vi "Rotation Matrix to Transform.vi"(1 "translation vector":dbl[](array[numeric]), 2 "rotation matrix":T1=[[1.0, 0.0, 0.0], [0.0, 1.0, 0.0], [0.0, 0.0, 1.0]]) -> (0 "transform":T1)   [LabVIEW 2017, in "NI_Kinematics.lvlib"]
doc: "Returns the transform that corresponds to the <B>rotation matrix</B> and <B>translation vector</B> you specify.\n\n<B>.m file:</B> r2t"
uses:
  <vilib>/robotics/Kinematics/NI_Kinematics.lvlib
  <vilib>/Analysis/Matrix/Datatypes/RealMatrix.ctl
  <vilib>/Analysis/Matrix/NI_Matrix.lvlib
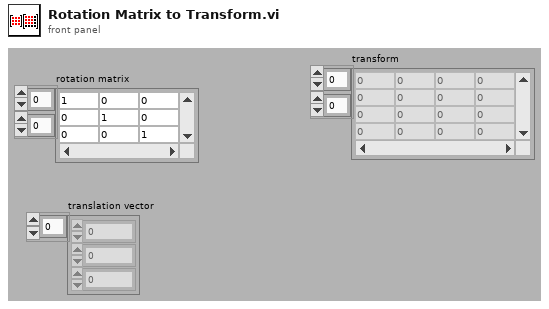
[diagram p1: front panel]
types:
  T1 = typedef "NI_Matrix.lvlib/RealMatrix.ctl" = dbl[][]
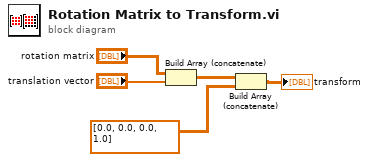
[diagram p0: block diagram]
diagram:
  n1 = Build Array (concatenate)("rotation matrix", "translation vector") -> (w1:T1)
  n2 = Build Array (concatenate)(w1, dbl[][] [[0.0, 0.0, 0.0, 1.0]] ("element")) -> (→"transform":T1)
